vi "Calculate Sample Buffer Size.vi"(10 "Reverse (F)":bool, 11 "Speed Multiplier":dbl format="%#_13g") -> (3 "Sample Size":i32)   [LabVIEW 2019, in "Audio Processing.lvlib"]
doc: "Calculate the size of the audio buffer based on the playback speed."
uses:
  Audio Processing.lvlib
  Globals.lvlibp/Constants.vi
  Globals.lvlibp
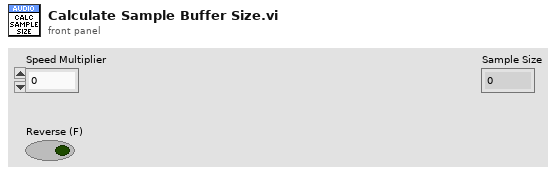
[diagram p1: front panel]
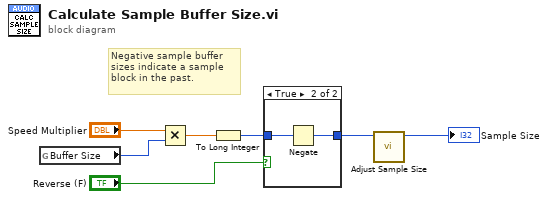
[diagram p0: block diagram]
diagram:
  # "Negative sample buffer sizes indicate a sample block in the past."
  n1 = global read "Constants.vi" "Buffer Size"() -> (w2:i32)
  n2 = Multiply(x="Speed Multiplier", y=w2) -> (x*y=w5:dbl)
  n3 = To Long Integer(number=w5) -> (32bit integer=w4:i32)
  n4 = case shown="True" "Reverse (F)" {
    tunnel: w4 -> [w8 w10]
    tunnel: [w8 w9] -> w3
    frame False {
    }
    frame True {
      n5 = Negate(x=w10) -> (-x=w9:i32)
    }
  }
  n6 = call "Adjust Sample Size.vi"("Sample Size In"=w3) -> ("Sample Size Out"=→"Sample Size":i32)  [unwired: 10 in]
